vi "hmi_cheesy_drive.vi"(7 "Turn Gains":T1={"Quickturn_Sens_Low"=1.2, "Quickturn_Sens_High"=1.0, "Speedturn_Sens_Low"=1.5, "Speedturn_Sens_High"=1.7}, 9 "Quick Turn":bool, 10 "Wheel":dbl, 11 "Throttle":dbl) -> (3 "Drive Data":cluster{"Left":dbl, "Right":dbl})   [LabVIEW 2013]
uses:
  Robot Global Data.vi
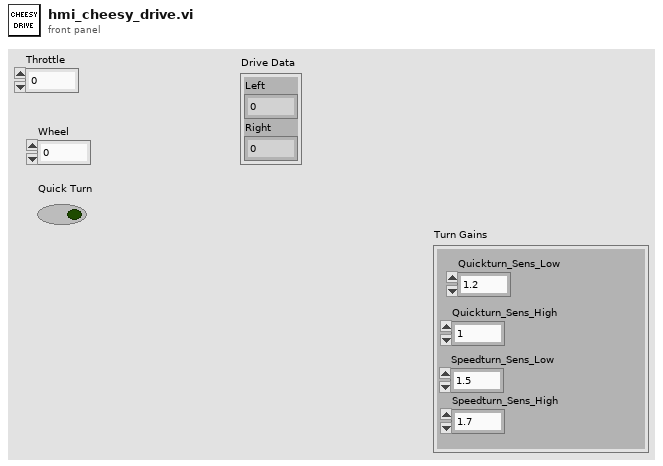
[diagram p1: front panel]
types:
  T1 = cluster{"Quickturn_Sens_Low":dbl, "Quickturn_Sens_High":dbl, "Speedturn_Sens_Low":dbl, "Speedturn_Sens_High":dbl}
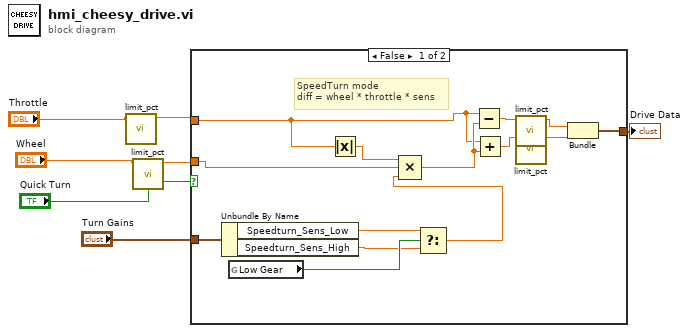
[diagram p0: block diagram]
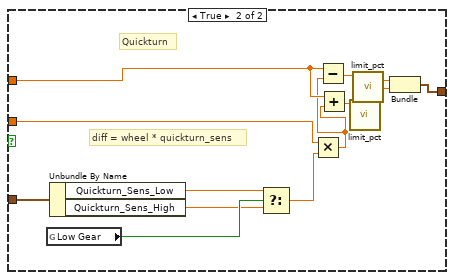
[diagram p2: hidden frame]
diagram:
  n1 = call "limit_pct.vi"("PCT"="Throttle") -> ("PCT Out"=w4:dbl)  [unwired: 10 in]
  n2 = call "limit_pct.vi"("PCT"="Wheel") -> ("PCT Out"=w2:dbl)  [unwired: 10 in]
  n3 = case shown="False" "Quick Turn" {
    tunnel: w2 -> [w21 w33]
    tunnel: w4 -> [w12 w32]
    tunnel: [w18 w30] -> w6
    tunnel: "Turn Gains" -> [w10 w24]
    frame False {
      # "SpeedTurn mode\ndiff = wheel * throttle * sens"
      n4 = Unbundle By Name(w10) -> ("Speedturn_Sens_Low"=w8:dbl, "Speedturn_Sens_High"=w9:dbl)
      n5 = global read "Robot Global Data.vi" "Low Gear"() -> (w11:bool)
      n6 = Absolute Value(x=w12) -> (abs(x)=w13:dbl)
      n7 = Select(t=w8, s=w11, f=w9) -> (s? t:f=w20:dbl)
      n8 = Compound Arithmetic op=MULTIPLY(w13, w21, w20) -> (w19:dbl)
      n9 = Subtract(x=w12, y=w19) -> (x-y=w16:dbl)
      n10 = Add(x=w12, y=w19) -> (x+y=w15:dbl)
      n11 = call "limit_pct.vi"("PCT"=w16) -> ("PCT Out"=w17:dbl)  [unwired: 10 in]
      n12 = call "limit_pct.vi"("PCT"=w15) -> ("PCT Out"=w14:dbl)  [unwired: 10 in]
      n13 = Bundle("PCT Out"=w17, "PCT Out"=w14) -> (w18:cluster{"PCT Out":dbl, "PCT Out":dbl})  [unwired: 1 in]
    }
    frame True {
      # "Quickturn"
      # "diff = wheel * quickturn_sens"
      n14 = global read "Robot Global Data.vi" "Low Gear"() -> (w25:bool)
      n15 = Unbundle By Name(w24) -> ("Quickturn_Sens_Low"=w23:dbl, "Quickturn_Sens_High"=w22:dbl)
      n16 = Select(t=w23, s=w25, f=w22) -> (s? t:f=w34:dbl)
      n17 = Multiply(x=w33, y=w34) -> (x*y=w31:dbl)
      n18 = Subtract(x=w32, y=w31) -> (x-y=w28:dbl)
      n19 = Add(x=w32, y=w31) -> (x+y=w26:dbl)
      n20 = call "limit_pct.vi"("PCT"=w26) -> ("PCT Out"=w27:dbl)  [unwired: 10 in]
      n21 = call "limit_pct.vi"("PCT"=w28) -> ("PCT Out"=w29:dbl)  [unwired: 10 in]
      n22 = Bundle("PCT Out"=w29, "PCT Out"=w27) -> (w30:cluster{"PCT Out":dbl, "PCT Out":dbl})  [unwired: 1 in]
    }
  }
  "Drive Data" <- w6
